vi "fetch-signal-data-from-dbc.vi"(8 "error in (no error)":errorcluster, 11 "signal.tag":string) -> (0 "error out":errorcluster, 3 "can.signal":T1={"Comment"="", "Byte Order"=125000, "Data Type"=0, "Number of Bits"=8, "Start Bit"=0, "Unit"="V", "Default Value"=0.0, "Minimum Value"=0.0, "Maximum Value"=256.0, "Scaling Offset"=0.0, "Scaling Factor"=1.0, "Signal name"="signal1"} {"Byte Order" items=["Little Endian", "Big Endian"]; "Data Type" items=["Signed", "Unsigned", "IEEE Float"]})   [LabVIEW 2015]
doc: "Use this template to build a VI to use as a subVI."
uses:
  controls/dbc-signal.ctl
  <vilib>/xnet/xnet.llb/XNET String To IO Name (Signal).vi
  <resource>/objmgr/xnet.rc
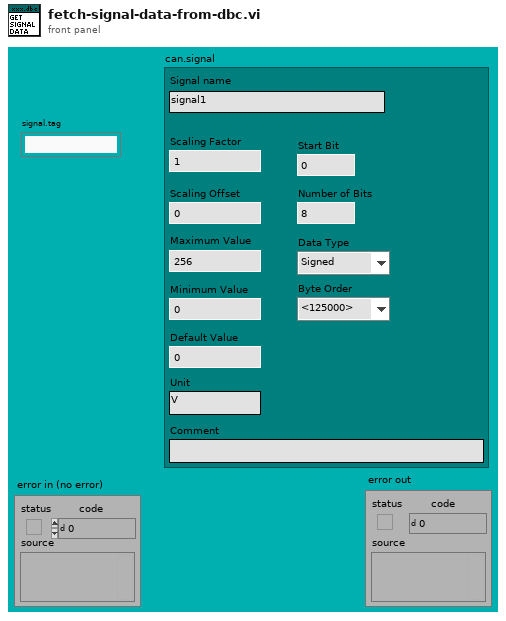
[diagram p1: front panel]
types:
  T1 = typedef "dbc-signal.ctl" = cluster{"Comment":string, "Byte Order":u32, "Data Type":u32, "Number of Bits":u32, "Start Bit":u32, "Unit":string, "Default Value":dbl, "Minimum Value":dbl, "Maximum Value":dbl, "Scaling Offset":dbl, "Scaling Factor":dbl, "Signal name":string}
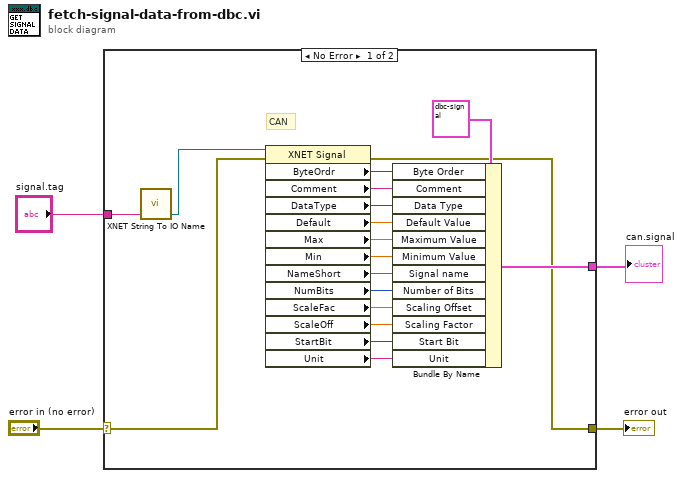
[diagram p0: block diagram]
diagram:
  n1 = case shown="No Error" "error in (no error)" {
    selector: "error in (no error)" -> [w19 w23]
    tunnel: [w5 w23] -> w3
    tunnel: "signal.tag" -> [w22 _]
    tunnel: [w20 _] -> w1
    frame No Error {
      # "CAN"
      n2 = call-poly <vilib>:"XNET String To IO Name.vi"("string"=w22) -> ("XNET Signal"=w21:refnum<k21>)  [unwired: 4 out]
      n3 = property class="XNET Signal"(reference=w21, error in=w19) -> (error out=w5:errorcluster, "ByteOrdr"=w17:u32, "Comment"=w16:string, "DataType"=w15:u32, "Default"=w14:dbl, "Max"=w13:dbl, "Min"=w12:dbl, "NameShort"=w11:string, "NumBits"=w10:u32, "ScaleFac"=w9:dbl, "ScaleOff"=w8:dbl, "StartBit"=w7:u32, "Unit"=w6:string)  [unwired: 1 out]
      n4 = Bundle By Name(cluster=T1 {"Comment"="", "Byte Order"=125000, "Data Type"=0, "Number of Bits"=8, "Start Bit"=0, "Unit"="V", "Default Value"=0.0, "Minimum Value"=0.0, "Maximum Value"=256.0, "Scaling Offset"=0.0, "Scaling Factor"=1.0, "Signal name"="signal1"} ("CAN Cluster"), "Byte Order"=w17, "Comment"=w16, "Data Type"=w15, "Default Value"=w14, "Maximum Value"=w13, "Minimum Value"=w12, "Signal name"=w11, "Number of Bits"=w10, "Scaling Offset"=w9, "Scaling Factor"=w8, "Start Bit"=w7, "Unit"=w6) -> (w20:T1)
    }
    frame Error {
    }
  }
  "error out" <- w3
  "can.signal" <- w1
